vi "ConfigureOphir.vi"(2 "error in (no error)":errorcluster, 3 "OphirRef In":T1) -> (0 "error out":errorcluster, 1 "OphirRef Out":T1)   [LabVIEW 2012]
uses:
  TypeDefs/OphirRef.ctl
  TypeDefs/FilterEnum.ctl
  TypeDefs/RangeEnum.ctl
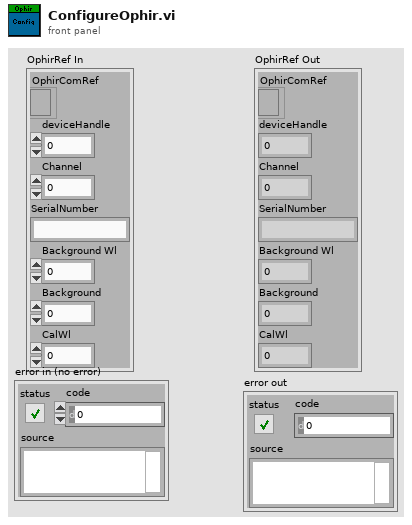
[diagram p1: front panel]
types:
  T1 = typedef "OphirRef.ctl" = cluster{"OphirComRef":refnum<k7>, "deviceHandle":i32, "Channel":i32, "SerialNumber":string, "Background Wl":dbl, "Background":dbl, "CalWl":dbl}
  T2 = typedef "RangeEnum.ctl" = enum16{"AUTO", "300mW", "30.0mW", "3.00mW", "300uW"}
  T3 = typedef "FilterEnum.ctl" = enum16{"OUT", "IN"}
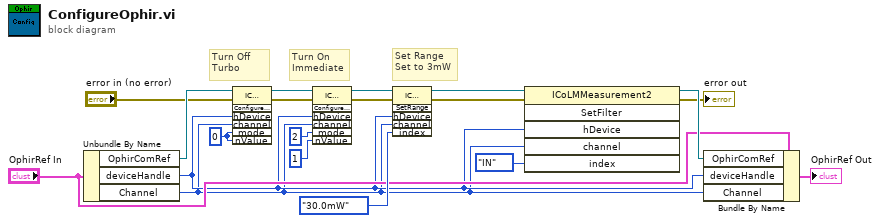
[diagram p0: block diagram]
diagram:
  w2 = 0 ("mode")
  # "Turn Off \nTurbo"
  # "Set Range\nSet to 3mW"
  # "Turn On \nImmediate"
  n1 = Unbundle By Name("OphirRef In") -> ("OphirComRef"=w7:refnum<k7>, "deviceHandle"=w4:i32, "Channel"=w3:i32)
  n2 = invoke class="ICoLMMeasurement2" method="ConfigureStreamMode"(reference=w7, error in="error in (no error)", "hDevice"=w4, "channel"=w3, "mode"=w2, "nValue"=w2) -> (reference out=w6:refnum<k7>, error out=w5:errorcluster)  [unwired: 1 in, 5 out]
  n3 = invoke class="ICoLMMeasurement2" method="ConfigureStreamMode"(reference=w6, error in=w5, "hDevice"=w4, "channel"=w3, "mode"=2, "nValue"=1) -> (reference out=w16:refnum<k7>, error out=w15:errorcluster)  [unwired: 1 in, 5 out]
  n4 = invoke class="ICoLMMeasurement2" method="SetRange"(reference=w16, error in=w15, "hDevice"=w4, "channel"=w3, "index"=RangeEnum."30.0mW" ("Range")) -> (reference out=w14:refnum<k7>, error out=w12:errorcluster)  [unwired: 1 in, 4 out]
  n5 = invoke class="ICoLMMeasurement2" method="SetFilter"(reference=w14, error in=w12, "hDevice"=w4, "channel"=w3, "index"=FilterEnum."IN" ("Filter")) -> (reference out=w11:refnum<k7>, error out=→"error out":errorcluster)  [unwired: 1 in, 4 out]
  n6 = Bundle By Name(cluster="OphirRef In", "OphirComRef"=w11, "deviceHandle"=w4, "Channel"=w3) -> (→"OphirRef Out":T1)
